vi "英维克空调解析.vi"(11 "数组":u16[](array[numeric]) format="%04xH") -> ()   [LabVIEW 2016, in "环境动力监测库.lvlib" / "空调库.lvlib"]
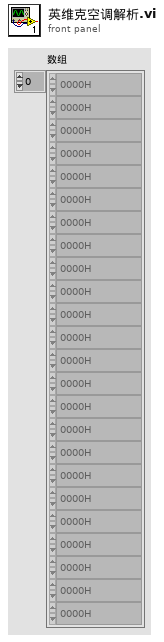
[diagram p1: front panel]
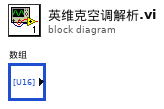
[diagram p0: block diagram]
diagram:
